vi "ReadOnePosition.vi"(8 "error in (no error)":errorcluster, 9 "Axis (1..4)":T1=1 items=["X"=1, "Y"=2, "Z"=3, "T"=4], 11 "VXMx2 in":refnum<class "VXMx2.lvclass">) -> (0 "error out":errorcluster, 1 "Position, eng units":dbl, 3 "VXMx2 out":refnum<class "VXMx2.lvclass">)   [LabVIEW 2018, in "VXMx2.lvclass"]
uses:
  VXMx2.lvclass
  <instrlib>/Velmex VXM/Public/VXM Axis.ctl
  VXMx2.lvclass/VXMx2.ctl
  <instrlib>/Velmex VXM/Velmex VXM.lvlib
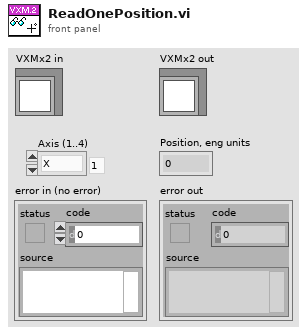
[diagram p1: front panel]
types:
  T1 = typedef "Velmex VXM.lvlib/VXM Axis.ctl" = u16
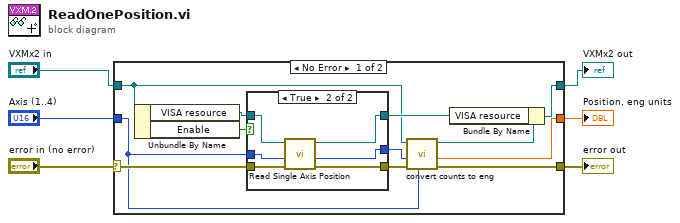
[diagram p0: block diagram]
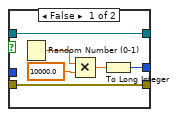
[diagram p2: hidden frame]
diagram:
  n1 = case shown="No Error" "error in (no error)" {
    selector: "error in (no error)" -> [w15 w32]
    tunnel: [w11 w32] -> w5
    tunnel: [w17 w31] -> w3
    tunnel: "VXMx2 in" -> [w10 w31]
    tunnel: "Axis (1..4)" -> [w13 _]
    tunnel: [w7 _] -> w1
    frame No Error {
      n2 = Unbundle By Name(w10) -> ("VISA resource"=w18:refnum<visa-resource-name>, "Enable"=w14:bool)
      n3 = case shown="True" w14 {
        tunnel: w13 -> [_ w30]
        tunnel: w18 -> [w20 w29]
        tunnel: [w20 w28] -> w16
        tunnel: w15 -> [w21 w27]
        tunnel: [w21 w26] -> w12
        tunnel: [w19 w25] -> w8
        frame False {
          n4 = Random Number (0-1)() -> (number: 0 to 1=w24:dbl)
          n5 = Multiply(x=w24, y=10000.0) -> (x*y=w22:dbl)
          n6 = To Long Integer(number=w22) -> (32bit integer=w19:i32)
        }
        frame True {
          n7 = call <instrlib>:"Read Single Axis Position.vi"("error in (no error)"=w27, "Axis (1..4)"=w30, "VISA resource name"=w29) -> ("error out"=w26:errorcluster, "Position, counts"=w25:i32, "VISA resource out"=w28:refnum<visa-resource-name>)  [unwired: 6 in]
        }
      }
      n8 = call "convert counts to eng.vi"("Axis (1..4)"=w13, "error in (no error)"=w12, "Position, counts"=w8, "VXMx2 in"=w10) -> ("error out"=w11:errorcluster, "Position, eng units"=w7:dbl, "VXMx2 out"=w9:refnum<class "VXMx2.lvclass">)  [unwired: 4 in, 1 out]
      n9 = Bundle By Name(cluster=w9, "VISA resource"=w16) -> (w17:refnum<class "VXMx2.lvclass">)
    }
    frame Error {
    }
  }
  "error out" <- w5
  "VXMx2 out" <- w3
  "Position, eng units" <- w1
